vi "Write Refresh Active Room Details Msg.vi"(10 "Rooms Manager UI.lvlib:Refresh Active Room Details Msg.lvclass":refnum<class "Refresh Active Room Details Msg.lvclass">, 11 "Rooms Manager UI in":refnum<class "Rooms Manager UI.lvclass">) -> (3 "Rooms Manager UI out":refnum<class "Rooms Manager UI.lvclass">)   [LabVIEW 2023, in "Rooms Manager UI.lvlib" / "Rooms Manager UI.lvclass"]
uses:
  Rooms Manager UI.lvclass
  Rooms Manager UI Messages/Refresh Active Room Details Msg/Refresh Active Room Details Msg.lvclass
  Rooms Manager UI.lvclass/Rooms Manager UI.ctl
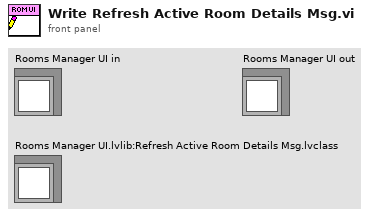
[diagram p1: front panel]
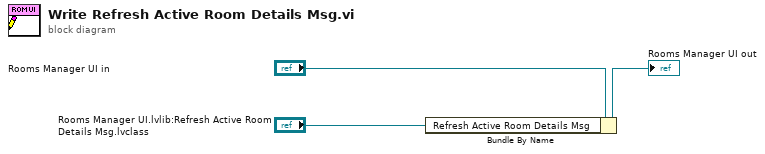
[diagram p0: block diagram]
diagram:
  n1 = Bundle By Name(cluster="Rooms Manager UI in", "Refresh Active Room Details Msg"="Rooms Manager UI.lvlib:Refresh Active Room Details Msg.lvclass") -> (→"Rooms Manager UI out":refnum<class "Rooms Manager UI.lvclass">)
